vi "CloseDotNetReferenceInArray.vi"(1 "Array Of .NET Refs":refnum<k24>[](array[refnum])) -> (0 "error out":errorcluster)   [LabVIEW 2011]
uses:
  D:/tsdev/Tests/LVBuildValidation/11.0/Automated/FlexLVAdapter30/Refnums/DotNetRefnum/LabviewDNTest.dll
  LabviewDNTest.dll
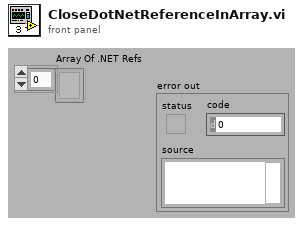
[diagram p1: front panel]
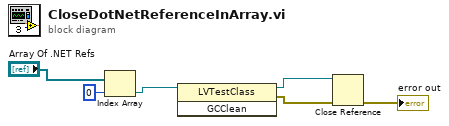
[diagram p0: block diagram]
diagram:
  n1 = Index Array(array="Array Of .NET Refs", index=0) -> (element=w3:refnum<k24>)
  n2 = invoke class="LVTestClass" method="GCClean"(reference=w3) -> (reference out=w2:refnum<k24>, error out=w1:errorcluster)  [unwired: 2 in, 1 out]
  n3 = Close Reference(reference=w2, error in (no error)=w1) -> (error out=→"error out":errorcluster)
